vi "Mangle VI Name (String)__ogtk.vi"(8 "error in (no error)":errorcluster, 10 "Namespace (\"\": don't mangle)":string, 11 "Name":string) -> (0 "error out":errorcluster, 3 "Mangled Name":string)   [LabVIEW 2020]
doc: "Mangles a VI's name by applying a <b>namespace string suffix</b>.\n<b>Name</b> may be a path or a string.\nFor example:\n\nName => \"Widget.vi\"\nNamespace => \"OpenG\"\nMangled Name => \"Widget__OpenG.vi\"\n\nName => \"Widget\"\nNamespace => \"OpenG\"\nMangled Name => \"Widget__OpenG\"\n\nName => \"Widget.vi\"\nNamespace => \"\" (Note: blank string means do not mangle)\nMangled Name => \"Widget.vi\""
uses:
  <userlib>/_OpenG.lib/file/file.llb/Strip Path Extension - String__ogtk.vi
panel:
  # "Mangle VI Name.vi\n\nMangles a VI's name using the namespace input.\n\nPlease visit http://www.OpenG.org to learn about the\nOpen Source LabVIEW software movement.\n\nNOTICE -- YOU MUST LEAVE THIS NOTICE IN PLACE.  PER THE TERMS OF THE LICENSE BELOW, YOU MAY SUBLICENSE THIS SOFTWARE \nIN ANY WAY THAT DOES NOT CONFLICT WITH THIS LICENSE.\n\n### BSD License (http://www.opensource.org/licenses/bsd-license.php) Begin ###\n \nCopyright (c) 2002-2004, Jim Kring <jim@jimkring.com>\n\nAll rights reserved.\n\nRedistribution and use in source and binary forms, with or without modification, are permitted provided that the following conditions are met:\n\n    * Redistributions of source code must retain the above copyright notice, this list of conditions and the following disclaimer.\n    * Redistributions in binary form must reproduce the above copyright notice, this list of conditions and the following disclaimer in the \n       documentation and/or other materials provided with the distribution.\n    * Neither the name of SciWare, James Kring, Inc., nor the names of its contributors may be used to endorse or promote products derived \n       from this software without specific prior written permission.\n\nTHIS SOFTWARE IS PROVIDED BY THE COPYRIGHT HOLDERS AND CONTRIBUTORS \"AS IS\" AND ANY EXPRESS OR IMPLIED WARRANTIES, \nINCLUDING, BUT NOT LIMITED TO, THE IMPLIED WARRANTIES OF MERCHANTABILITY AND FITNESS FOR A PARTICULAR PURPOSE ARE \nDISCLAIMED. IN NO EVENT SHALL THE COPYRIGHT OWNER OR CONTRIBUTORS BE LIABLE FOR ANY DIRECT, INDIRECT, INCIDENTAL,\n SPECIAL, EXEMPLARY, OR CONSEQUENTIAL DAMAGES (INCLUDING, BUT NOT LIMITED TO, PROCUREMENT OF SUBSTITUTE GOODS OR \nSERVICES; LOSS OF USE, DATA, OR PROFITS; OR BUSINESS INTERRUPTION) HOWEVER CAUSED AND ON ANY THEORY OF LIABILITY, \nWHETHER IN CONTRACT, STRICT LIABILITY, OR TORT (INCLUDING NEGLIGENCE OR OTHERWISE) ARISING IN ANY WAY OUT OF THE USE \nOF THIS SOFTWARE, EVEN IF ADVISED OF THE POSSIBILITY OF SUCH DAMAGE.\n\n### BSD License End ###"
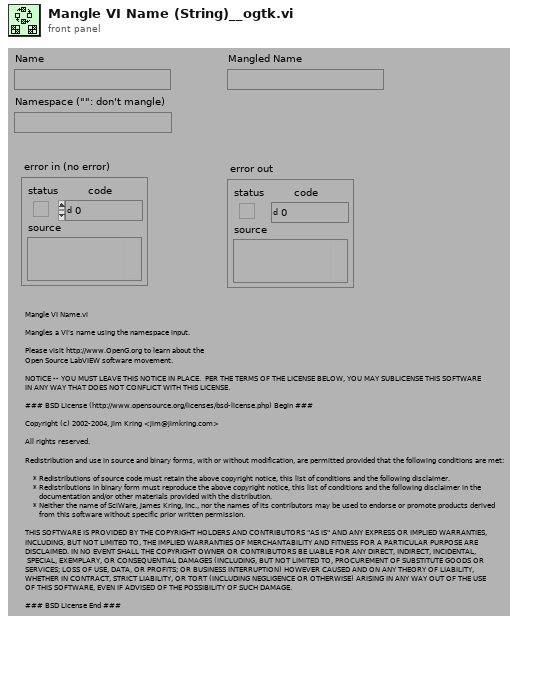
[diagram p1: front panel]
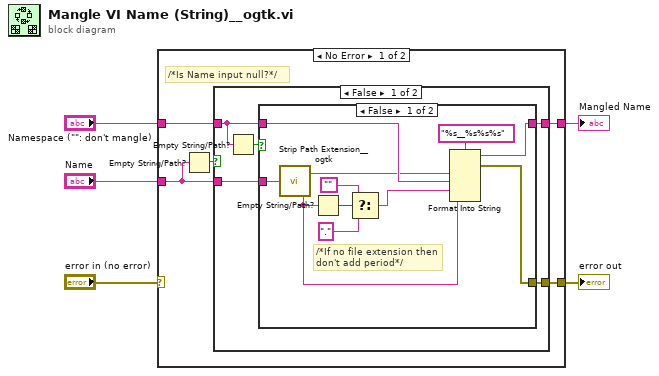
[diagram p0: block diagram]
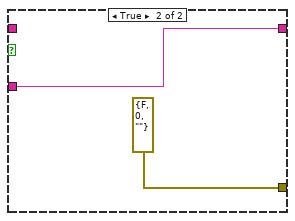
[diagram p2: hidden frame]
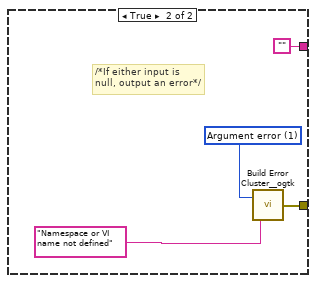
[diagram p3: hidden frame]
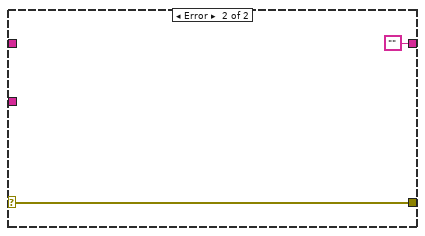
[diagram p4: hidden frame]
diagram:
  n1 = case shown="No Error" "error in (no error)" {
    selector: "error in (no error)" -> [_ w34]
    tunnel: [w10 ""] -> w5
    tunnel: "Name" -> [w9 _]
    tunnel: "Namespace (\"\": don't mangle)" -> [w8 _]
    tunnel: [w7 w34] -> w1
    frame No Error {
      # "/*Is Name input null?*/"
      n2 = Empty String/Path?(string/path=w9) -> (empty?=w6:bool)
      n3 = case shown="False" w6 {
        tunnel: w9 -> [w13 _]
        tunnel: w8 -> [w12 _]
        tunnel: [w15 ""] -> w10
        tunnel: [w14 w31] -> w7
        frame False {
          n4 = Empty String/Path?(string/path=w12) -> (empty?=w11:bool)
          n5 = case shown="False" w11 {
            tunnel: w12 -> [w26 _]
            tunnel: [w20 w28] -> w15
            tunnel: [w24 errorcluster {"status"=FALSE, "code"=0, "source"=""} ("error IO")] -> w14
            tunnel: w13 -> [w23 w28]
            frame False {
              # "/*If no file extension then don't add period*/"
              n6 = call-poly <userlib>:"Strip Path Extension__ogtk.vi"("path"=w23) -> ("root"=w22:string, "extension"=w17:string)
              n7 = Empty String/Path?(string/path=w17) -> (empty?=w21:bool)
              n8 = Select(t="", s=w21, f=".") -> (s? t:f=w18:string)
              n9 = Format Into String(format string="%s__%s%s%s" ("Format String"), w22, w26, w18, w17) -> (resulting string=w20:string, error out=w24:errorcluster)  [unwired: 2 in]
            }
            frame True {
            }
          }
        }
        frame True {
          w30 = 1 items=["No error", "Argument error", "Memory is full", "Out of zone", "End of file", "File already open", "Generic file I/O error", "File not found", "File permission error", "Disk is full", "Duplicate path", "Too many files open", "System feature not enabled", "Resource file not found", "Cannot add resource", "Resource not found", "Image not found", "Image memory error", "Pen does not exist", "Config type invalid", "Config token not found", "Config parse error", "Config memory error", "Bad external code format", "Bad external code offset", "External code not present", "Null window", "Destroy window error", "Null menu", "Print aborted", "Bad print record", "Print driver error", "Windows error during printing", "Memory error during printing", "Print dialog error", "Generic print error", "Invalid device refnum", "Device not found", "Device parameter error", "Device unit error", "Cannot open device", "Device call aborted", "Generic error", "Cancelled by user", "Object ID too low", "Object ID too high", "Object not in heap", "Unknown heap", "Unknown object (invalid DefProc)", "Unknown object (DefProc not in table)", "Message out of range", "Invalid (null) method", "Unknown message", "Manager call not supported", "Bad address", "Network operation in progress", "Network operation timed out", "Connection is busy", "Network attribute not supported", "Network error", "Address in use", "System out of memory", "Connection aborted", "Connection refused", "Not connected", "Already connected", "Connection closed", "Initialization error (interapplication manager)", "Bad occurrence", "Wait on unbound occurrence handler", "Occurrence queue overflow", "Datalog type conflict", "Unused", "Unrecognized type (interapplication manager)", "Memory corrupt", "Failed to make temporary DLL", "Old CIN version", "Drag socket not found", "Failed to load drop-object", "Failed to register OLE object", "Failed to release OLE object", "Format specifier type mismatch", "Unknown format specifier", "Too few format specifiers", "Too many format specifiers", "Scan failed", "Newer CIN version", "Error converting to variant", "Runtime menu error", "Password tampered", "Variant attribute not found", "Incompatible variant data type", "Event data is not available", "Event Store is not present", "Occurrence is not found", "Event Queue is not created", "Event info is not available", "Refnum passed is NULL", "Error retrieving Class GUID", "Error retrieving CoClass GUID", "Error retrieving TypeLib GUID.", "Bad built application magic bytes.", "Specific driver is different from the specific driver associated with the Logical Name.", "There is no session opened to the class driver.", "Max Error", "MAX - Error with config objects", "MAX - Error loading configuration", "MAX - Group not supported"]
          # "/*If either input is null, output an error*/"
          n10 = call <userlib>:"Build Error Cluster__ogtk.vi"("String to Prepend to source (\"\")"="Namespace or VI name not defined" ("String to Prepend to source (\"\")"), "code"=w30) -> ("error out"=w31:errorcluster)
        }
      }
    }
    frame Error {
    }
  }
  "Mangled Name" <- w5
  "error out" <- w1
